vi "Write Main Config.vi"(8 "error in (no error)":errorcluster, 9 "Config":string, 10 "Main Config Path":path, 11 "System Config Module in":refnum<class "System Config Module.lvclass">) -> (0 "error out":errorcluster, 3 "System Config Module out":refnum<class "System Config Module.lvclass">)   [LabVIEW 2020, in "Volatus.lvlib" / "System Config Module.lvclass"]
uses:
  System Config Module.lvclass
  System Config Module.lvclass/System Config Module.ctl
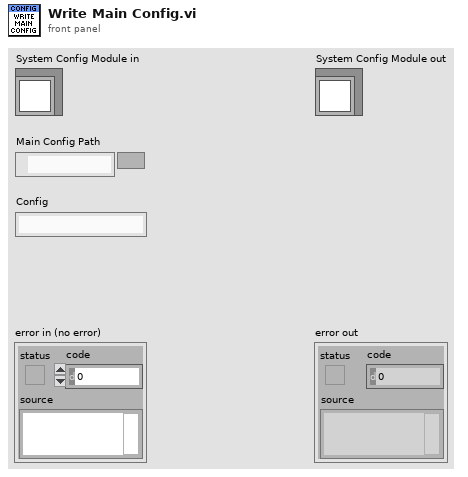
[diagram p1: front panel]
types:
  T1 = enum16{"open", "replace", "create", "open or create", "replace or create", "replace or create with confirmation"}
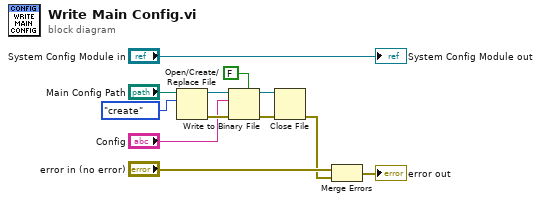
[diagram p0: block diagram]
diagram:
  n1 = Open/Create/Replace File(file path (use dialog)="Main Config Path", operation (0:open)=T1."create") -> (refnum out=w8:refnum<file>, error out=w7:errorcluster)  [unwired: 4 in, 1 out]
  n2 = Write to Binary File(file (use dialog)=w8, data="Config", error in=w7, 5:FALSE ("prepend array or string size? (T)")) -> (refnum out=w3:refnum<file>, error out=w4:errorcluster)  [unwired: 2 in, 1 out]
  n3 = Close File(refnum=w3, error in=w4) -> (error out=w1:errorcluster)  [unwired: 1 out]
  n4 = Merge Errors("error in (no error)", w1) -> (→"error out":errorcluster)
  "System Config Module out" <- "System Config Module in"
